vi "Generic File Dialog.vi"(6 "Selection mode":enum16{"New", "Existing", "New or Existing"}(ring), 8 "error in (no error)":errorcluster, 10 "pattern (all files)":string="*ini", 11 "Parameter Generic File in":refnum<class "Parameter Generic File.lvclass">) -> (0 "error out":errorcluster, 3 "Parameter Generic File out":refnum<class "Parameter Generic File.lvclass">)   [LabVIEW 2019, in "CD Parameter Manager API.lvlib" / "Parameter Generic File.lvclass"]
uses:
  Parameter Generic File.lvclass
  Parameter Generic File.lvclass/Parameter Generic File.ctl
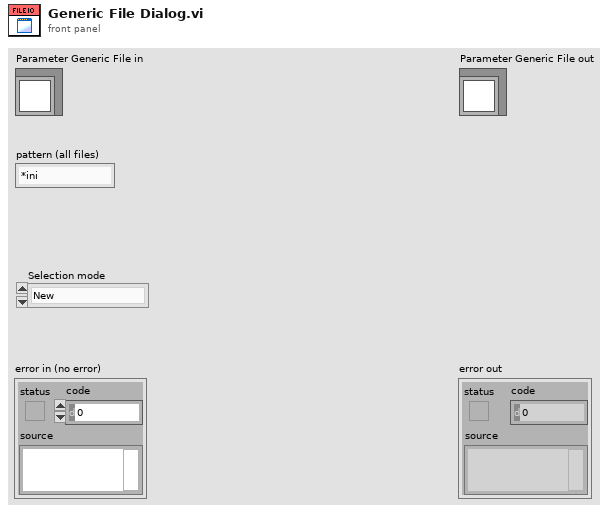
[diagram p1: front panel]
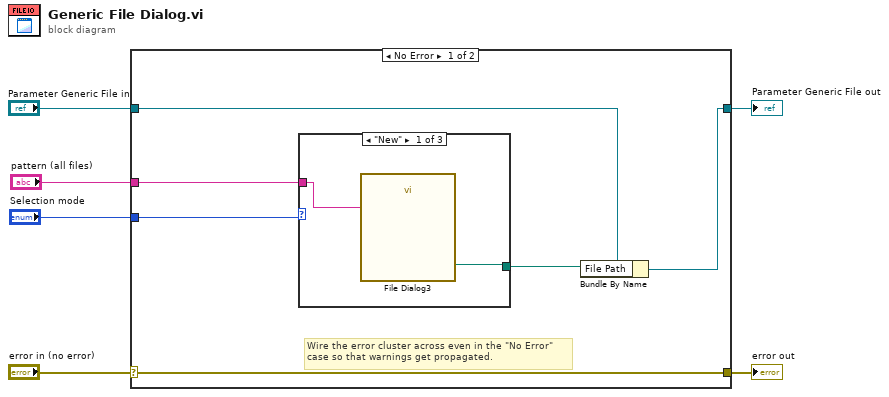
[diagram p0: block diagram]
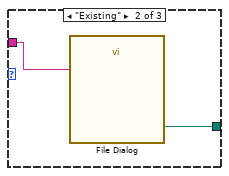
[diagram p2: hidden frame]
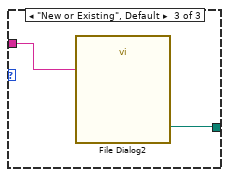
[diagram p3: hidden frame]
diagram:
  n1 = case shown="No Error" "error in (no error)" {
    selector: "error in (no error)" -> [w12 w20]
    tunnel: [w12 w20] -> w5
    tunnel: [w8 w19] -> w3
    tunnel: "Parameter Generic File in" -> [w9 w19]
    tunnel: "Selection mode" -> [w11 _]
    tunnel: "pattern (all files)" -> [w10 _]
    frame No Error {
      # "Wire the error cluster across even in the \"No Error\"\ncase so that warnings get propagated."
      n2 = case shown="\"New\"" w11 {
        tunnel: w10 -> [w14 w16 w18]
        tunnel: [w13 w15 w17] -> w7
        frame "New" {
          n3 = call "File Dialog3"("pattern (all files)"=w14) -> ("selected path"=w13:path)  [unwired: 11 in, 3 out]
        }
        frame "Existing" {
          n4 = call "File Dialog"("pattern (all files)"=w16) -> ("selected path"=w15:path)  [unwired: 11 in, 3 out]
        }
        frame "New or Existing", Default {
          n5 = call "File Dialog2"("pattern (all files)"=w18) -> ("selected path"=w17:path)  [unwired: 11 in, 3 out]
        }
      }
      n6 = Bundle By Name(cluster=w9, "File Path"=w7) -> (w8:refnum<class "Parameter Generic File.lvclass">)
    }
    frame Error {
    }
  }
  "error out" <- w5
  "Parameter Generic File out" <- w3
